vi "loadDataNodeEnd.vi"(8 "error in (no error)":errorcluster, 10 "XML Refnum in":refnum<file>, 11 "Channel in":refnum<class "Channel.lvclass">) -> (0 "error out":errorcluster, 2 "XML Refnum out":refnum<file>, 3 "Channel out":refnum<class "Channel.lvclass">)   [LabVIEW 2013, in "Channel.lvclass"]
doc: "Part of the file loading process. Occurs at the end of a node being loaded. Includes checking the end of the tag which has the format </tag>."
uses:
  Channel.lvclass
  xCE/xceDataNode/xceDataNode.lvclass
  XML Parser/XML Parser.lvclass
panel:
  out "Comment":string
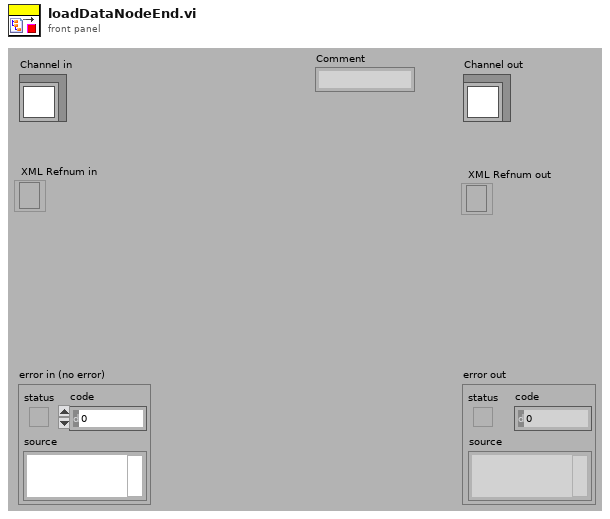
[diagram p1: front panel]
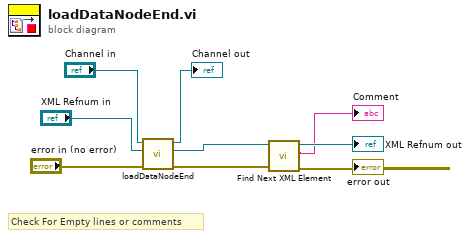
[diagram p0: block diagram]
diagram:
  # "Check For Empty lines or comments"
  n1 = call-parent "loadDataNodeEnd.vi"("error in (no error)"="error in (no error)", "XML Refnum in"="XML Refnum in", "xceDataNode in"="Channel in") -> ("error out"=w5:errorcluster, "XML Refnum out"=w4:refnum<file>, "xceDataNode out"=→"Channel out":refnum<class "Channel.lvclass">)  [unwired: 6 in]
  n2 = call "Find Next XML Element.vi"("error in (no error)"=w5, "XML Fine In"=w4) -> ("error out"=→"error out":errorcluster, "Comment"=→"Comment":string, "XML Fine Out"=→"XML Refnum out":refnum<file>)  [unwired: 7 in]
